vi "1_13_matrix_matrix_multiply.vi"(1 "p":i32, 3 "n":i32, 4 "m":i32, 5 "B":fxp<+/-,1,13>[](array[numeric]), 6 "A":fxp<+/-,1,13>[](array[numeric])) -> (0 "C":fxp<+/-,1,13>[](array[numeric]))   [LabVIEW 2020]
panel:
  in  "accum":fxp<+/-,1,13>
  in  "C_type":fxp<+/-,1,13>
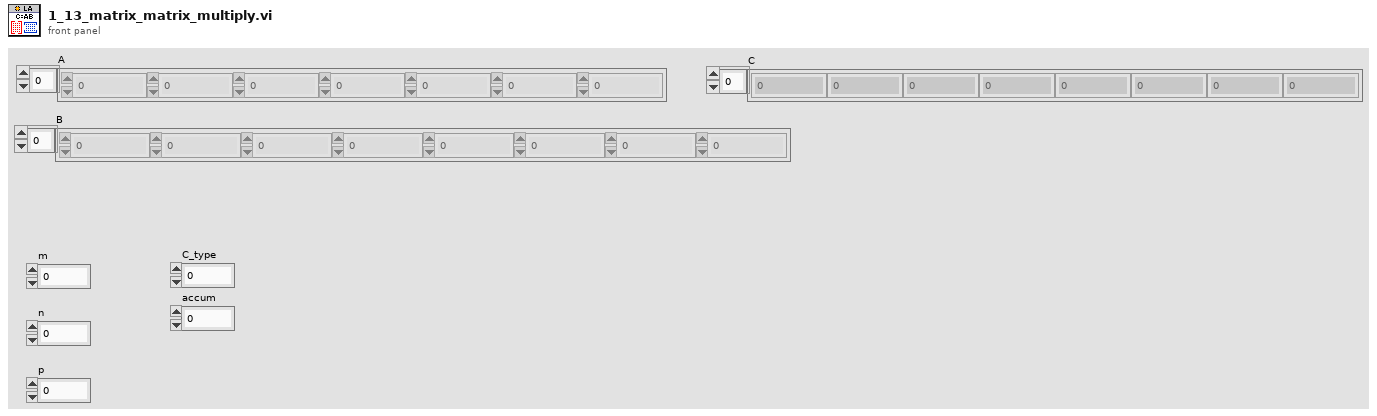
[diagram p1: front panel]
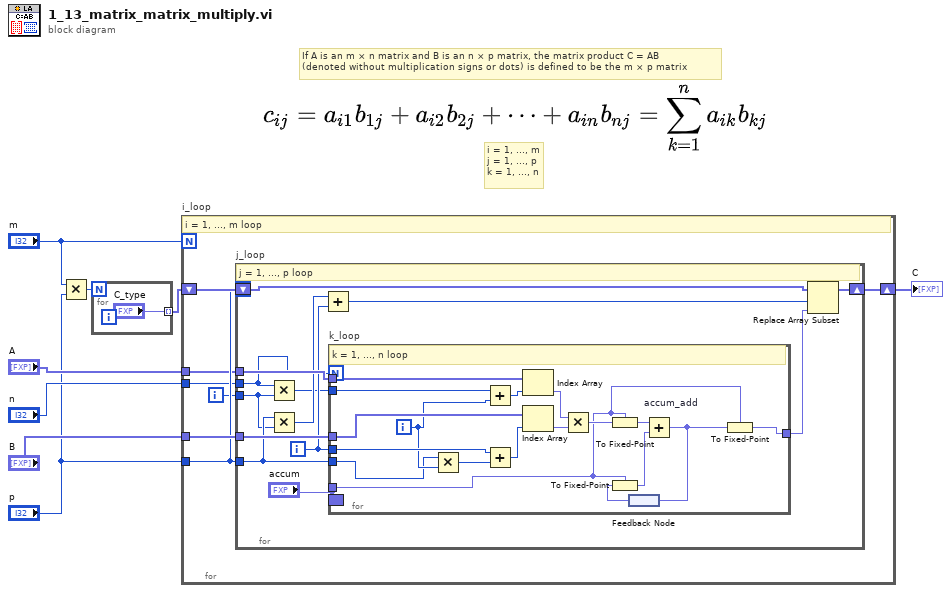
[diagram p0: block diagram]
diagram:
  # "If A is an m × n matrix and B is an n × p matrix, the matrix product C = AB \n(denoted without multiplication signs or dots) is defined to be the m × p matrix"
  # "i = 1, ..., m\nj = 1, ..., p\nk = 1, ..., n"
  n1 = Multiply(x="m", y="p") -> (x*y=w4:i32)
  n2 = for {
    N: w4 -> [_]
    tunnel: ["C_type"] -> w1 mode=indexing
  }
  n3 = for "i_loop" {
    N: "m" -> [_]
    tunnel: "B" -> [w16]
    tunnel: "p" -> [w13]
    tunnel: "A" -> [w12]
    tunnel: "n" -> [w11]
    shift-right: [w14] -> w6
    shift-left: w1 -> [w15]
    i -> [w10]
    # "i = 1, ..., m loop"
    n4 = for "j_loop" {
      N: w13 -> [_]
      tunnel: w12 -> [w29]
      tunnel: w16 -> [w28]
      tunnel: w13 -> [w20]
      shift-right: [w26] -> w14
      shift-left: w15 -> [w27]
      tunnel: w11 -> [w19]
      tunnel: w10 -> [w18]
      i -> [w23]
      # "j = 1, ..., p loop"
      n5 = Multiply(x=w19, y=w18) -> (x*y=w21:i32)
      n6 = Multiply(x=w20, y=w18) -> (x*y=w22:i32)
      n7 = Add(x=w22, y=w23) -> (x+y=w24:i32)
      n8 = for "k_loop" {
        N: w19 -> [_]
        tunnel: w29 -> [w47]
        tunnel: w21 -> [w37]
        tunnel: w28 -> [w46]
        tunnel: w23 -> [w43]
        tunnel: [w31] -> w25
        tunnel: w20 -> [w41]
        border: "accum" -> [_]
        tunnel: "accum" -> [w30]
        i -> [w42]
        # "k = 1, ..., n loop"
        n9 = Multiply(x=w41, y=w42) -> (x*y=w40:i32)
        n10 = Add(x=w37, y=w42) -> (x+y=w38:i32)
        n11 = Add(x=w43, y=w40) -> (x+y=w39:i32)
        n12 = Index Array(array=w47, index=w38) -> (element=w45:fxp<+/-,1,13>)
        n13 = Index Array(array=w46, index=w39) -> (element=w44:fxp<+/-,1,13>)
        n14 = Multiply(x=w45, y=w44) -> (x*y=w34:fxp<+,1,25>)
        n15 = To Fixed-Point(fixed-point type=w30, number=w34) -> (fixed-point=w33:fxp<+/-,1,13>)
        n16 = feedback #1() -> (w36:fxp<+/-,2,14>)
        n17 = To Fixed-Point(fixed-point type=w30, number=w36) -> (fixed-point=w35:fxp<+/-,1,13>)
        n18 = Add "accum_add"(x=w33, y=w35) -> (x+y=w32:fxp<+/-,2,14>)
        n19 = feedback-in #1(w32) -> ()
        n20 = To Fixed-Point(fixed-point type=w30, number=w32) -> (fixed-point=w31:fxp<+/-,1,13>)
      }
      n21 = Replace Array Subset(array=w27, new element=w25, index=w24) -> (w26:fxp<+/-,1,13>[])
    }
  }
  "C" <- w6
